vi "SRU2P（Boolean）.vi"(5 "初始值":bool, 6 "复位":bool, 7 "启用（T）":bool=TRUE, 9 "Yi":bool, 10 "Xi":bool) -> (1 "Yi-1":bool, 2 "Xi-1":bool)   [LabVIEW 2012]
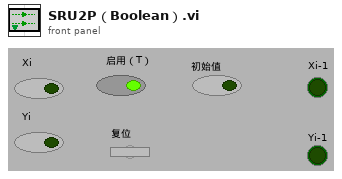
[diagram p1: front panel]
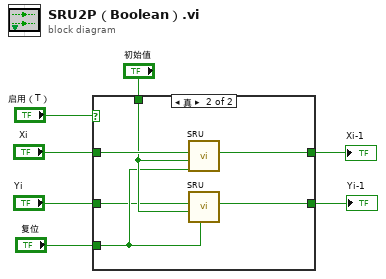
[diagram p0: block diagram]
diagram:
  n1 = case shown="真" "启用（T）" {
    tunnel: "复位" -> [_ w13]
    tunnel: "Xi" -> [w9 w15]
    tunnel: [w9 w12] -> w5
    tunnel: "初始值" -> [_ w14]
    tunnel: [w8 w11] -> w2
    tunnel: "Yi" -> [w8 w10]
    frame False {
    }
    frame True {
      n2 = call-poly "SRU.vi"("复位"=w13, "初始值"=w14, "输入"=w15) -> ("上次值"=w12:bool)  [unwired: 6 in, 2 out]
      n3 = call-poly "SRU.vi"("复位"=w13, "初始值"=w14, "输入"=w10) -> ("上次值"=w11:bool)  [unwired: 6 in, 2 out]
    }
  }
  "Xi-1" <- w5
  "Yi-1" <- w2
